vi "8.1.SSD1306_64x48_Example.vi"   [LabVIEW 2014]
uses:
  QwaveSys_Interface/QwaveSys_Interface.lvlib
  <vilib>/Aledyne-TSXperts/Arduino Compatible Compiler for LabVIEW/Arduino Compatible Compiler for LabVIEW.lvlib
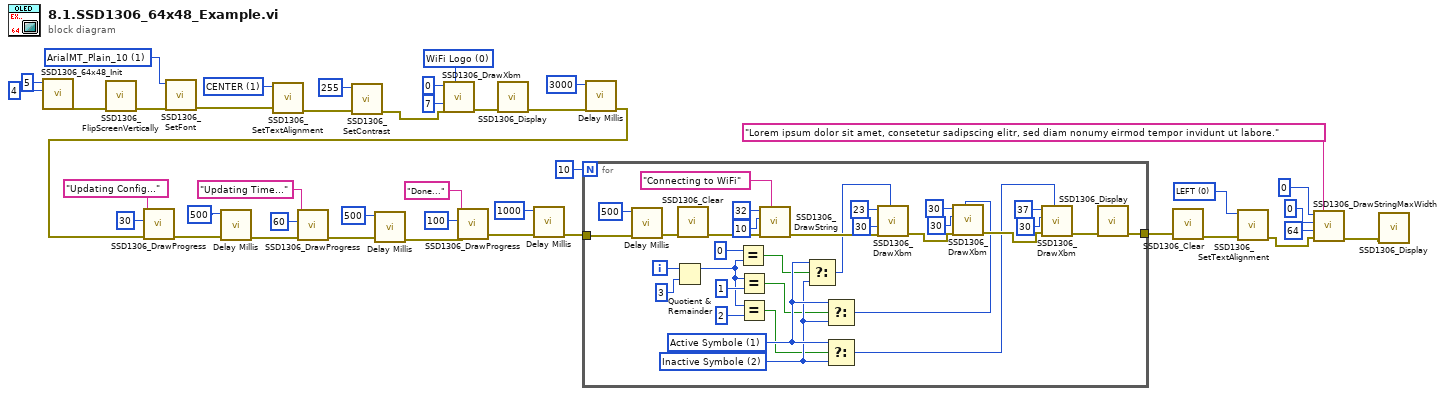
[diagram p0: block diagram]
diagram:
  w6 = u16 0 items=["WiFi Logo", "Active Symbole", "Inactive Symbole"] ("xbm")
  w11 = u16 0 items=["LEFT", "CENTER", "RIGHT"] ("alignment")
  w39 = u16 1 items=["LEFT", "CENTER", "RIGHT"] ("alignment")
  w37 = u16 1 items=["Crushed_Plain_36", "ArialMT_Plain_10", "ArialMT_Plain_16", "ArialMT_Plain_24"] ("Font")
  n1 = call "SSD1306_64x48_Init.vi"("SDA"=u8 4, "SCL"=u8 5) -> ("error out"=w1:errorcluster)  [unwired: 9 in]
  n2 = call "SSD1306_FlipScreenVertically.vi"("error in (no error)"=w1) -> ("error out"=w2:errorcluster)  [unwired: 10 in]
  n3 = call "SSD1306_SetFont.vi"("error in (no error)"=w2, "Font"=w37) -> ("error out"=w40:errorcluster)  [unwired: 9 in]
  n4 = call "SSD1306_SetTextAlignment.vi"("error in (no error)"=w40, "alignment"=w39) -> ("error out"=w38:errorcluster)  [unwired: 9 in]
  n5 = call "SSD1306_SetContrast.vi"("error in (no error)"=w38, "contrast"=u8 255) -> ("error out"=w35:errorcluster)  [unwired: 9 in]
  n6 = call "SSD1306_DrawXbm.vi"("xbm"=w6, "error in (no error)"=w35, "y"=u8 7, "x"=u8 0) -> ("error out"=w4:errorcluster)  [unwired: 7 in]
  n7 = call "SSD1306_Display.vi"("error in (no error)"=w4) -> ("error out"=w3:errorcluster)  [unwired: 10 in]
  n8 = call <vilib>:"Delay Millis.vi"("error in (no error)"=w3, "delay"=u32 3000) -> ("error out"=w22:errorcluster)  [unwired: 9 in]
  n9 = call "SSD1306_DrawProgress.vi"("error in (no error)"=w22, "percentage"=u8 30 ("%"), "String"="Updating Config...") -> ("error out"=w25:errorcluster)  [unwired: 8 in]
  n10 = call <vilib>:"Delay Millis.vi"("error in (no error)"=w25, "delay"=u32 500) -> ("error out"=w23:errorcluster)  [unwired: 9 in]
  n11 = call "SSD1306_DrawProgress.vi"("error in (no error)"=w23, "percentage"=u8 60 ("%"), "String"="Updating Time...") -> ("error out"=w33:errorcluster)  [unwired: 8 in]
  n12 = call <vilib>:"Delay Millis.vi"("error in (no error)"=w33, "delay"=u32 500) -> ("error out"=w32:errorcluster)  [unwired: 9 in]
  n13 = call "SSD1306_DrawProgress.vi"("error in (no error)"=w32, "percentage"=u8 100 ("%"), "String"="Done...") -> ("error out"=w19:errorcluster)  [unwired: 8 in]
  n14 = call <vilib>:"Delay Millis.vi"("error in (no error)"=w19, "delay"=u32 1000) -> ("error out"=w20:errorcluster)  [unwired: 9 in]
  n15 = for {
    N: 10 -> [_]
    tunnel: [w46] -> w14
    tunnel: w20 -> [w45]
    i -> [w74]
    w54 = u16 2 items=["WiFi Logo", "Active Symbole", "Inactive Symbole"] ("xbm")
    w55 = u16 1 items=["WiFi Logo", "Active Symbole", "Inactive Symbole"] ("xbm")
    n16 = call <vilib>:"Delay Millis.vi"("error in (no error)"=w45, "delay"=u32 500) -> ("error out"=w72:errorcluster)  [unwired: 9 in]
    n17 = Quotient & Remainder(x=w74, y=3) -> (x-y*floor(x/y)=w44:i32)  [unwired: 1 out]
    n18 = call "SSD1306_Clear.vi"("error in (no error)"=w72) -> ("error out"=w69:errorcluster)  [unwired: 10 in]
    n19 = Equal?(x=0, y=w44) -> (x = y?=w53:bool)
    n20 = Equal?(x=w44, y=1) -> (x = y?=w52:bool)
    n21 = Equal?(x=w44, y=2) -> (x = y?=w51:bool)
    n22 = call "SSD1306_DrawString.vi"("String"="Connecting to WiFi", "error in (no error)"=w69, "y"=u8 10, "x"=u8 32) -> ("error out"=w68:errorcluster)  [unwired: 7 in]
    n23 = Select(t=w55, s=w53, f=w54) -> (s? t:f=w49:u16)
    n24 = Select(t=w55, s=w52, f=w54) -> (s? t:f=w50:u16)
    n25 = Select(t=w55, s=w51, f=w54) -> (s? t:f=w48:u16)
    n26 = call "SSD1306_DrawXbm.vi"("xbm"=w49, "error in (no error)"=w68, "y"=u8 30, "x"=u8 23) -> ("error out"=w60:errorcluster)  [unwired: 7 in]
    n27 = call "SSD1306_DrawXbm.vi"("xbm"=w50, "error in (no error)"=w60, "y"=u8 30, "x"=u8 30) -> ("error out"=w59:errorcluster)  [unwired: 7 in]
    n28 = call "SSD1306_DrawXbm.vi"("xbm"=w48, "error in (no error)"=w59, "y"=u8 30, "x"=u8 37) -> ("error out"=w47:errorcluster)  [unwired: 7 in]
    n29 = call "SSD1306_Display.vi"("error in (no error)"=w47) -> ("error out"=w46:errorcluster)  [unwired: 10 in]
  }
  n30 = call "SSD1306_Clear.vi"("error in (no error)"=w14) -> ("error out"=w13:errorcluster)  [unwired: 10 in]
  n31 = call "SSD1306_SetTextAlignment.vi"("error in (no error)"=w13, "alignment"=w11) -> ("error out"=w12:errorcluster)  [unwired: 9 in]
  n32 = call "SSD1306_DrawStringMaxWidth.vi"("String"="Lorem ipsum dolor sit amet, consetetur sadipscing elitr, sed diam nonumy eirmod tempor invidunt ut labore.", "error in (no error)"=w12, "max line width"=u8 64, "y"=u8 0, "x"=u8 0) -> ("error out"=w15:errorcluster)  [unwired: 6 in]
  n33 = call "SSD1306_Display.vi"("error in (no error)"=w15) -> ()  [unwired: 10 in, 1 out]
